vi "Transport Data.vi"(8 "error in (no error)":errorcluster, 9 "Publication Time (Get Time)":timestamp, 10 "Value":variant, 11 "ITransport in":refnum<class "ITransport.lvclass">) -> (0 "error out":errorcluster, 3 "ITransport out":refnum<class "ITransport.lvclass">)   [LabVIEW 2018, in "MVA Framework.lvlib" / "ITransport.lvclass"]
doc: "传输数据"
uses:
  ITransport.lvclass
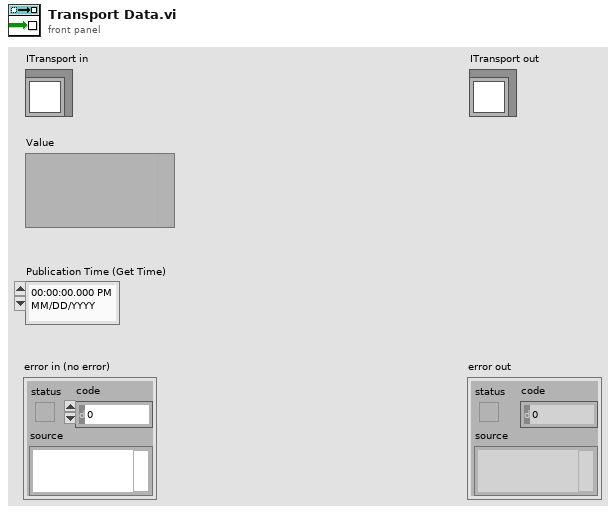
[diagram p1: front panel]
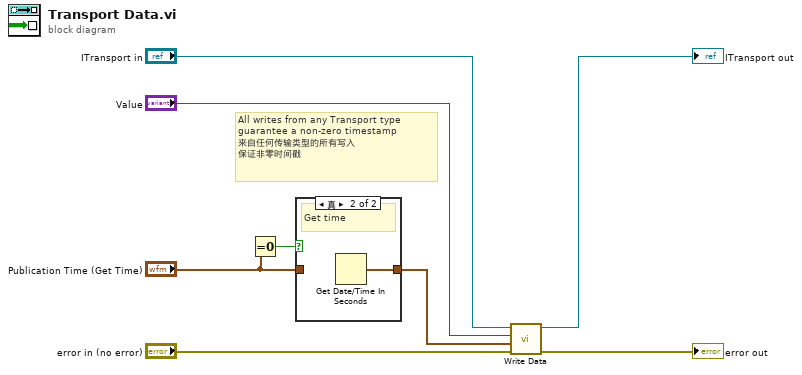
[diagram p0: block diagram]
diagram:
  # "All writes from any Transport type\nguarantee a non-zero timestamp\n来自任何传输类型的所有写入\n保证非零时间戳"
  n1 = Equal To 0?(x="Publication Time (Get Time)") -> (x = 0?=w4:bool)
  n2 = case shown="真" w4 {
    tunnel: "Publication Time (Get Time)" -> [w9 _]
    tunnel: [w9 w10] -> w1
    frame False {
      # "Use input time"
    }
    frame True {
      # "Get time"
      n3 = Get Date/Time In Seconds() -> (seconds since 1Jan1904=w10:timestamp)
    }
  }
  n4 = call-dynamic "Write Data.vi"("error in (no error)"="error in (no error)", "Publication Time"=w1, "Value"="Value", "ITransport in"="ITransport in") -> ("error out"=→"error out":errorcluster, "ITransport out"=→"ITransport out":refnum<class "ITransport.lvclass">)  [unwired: 6 in]
